vi "COM.vi"() -> ()   [LabVIEW 2013]
uses:
  <vilib>/Utility/file.llb/Write To Spreadsheet File (DBL).vi
panel:
  in  "Відстань \nреагування":dbl=30.0
  out "OloLo":bool
  out "Відстань в см.":dbl
  in  "Шлях для збереження даних в файл":path=path "C:/ULTRA/COM/first.csv"
  out "Посилка":i32
  in  "stop":bool
  out "Отриманий текст":string
  in  "Вибір порта для\n отримання даних":refnum<visa-resource-name>
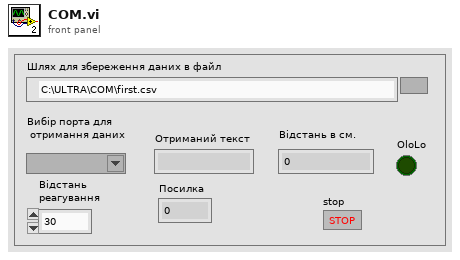
[diagram p1: front panel]
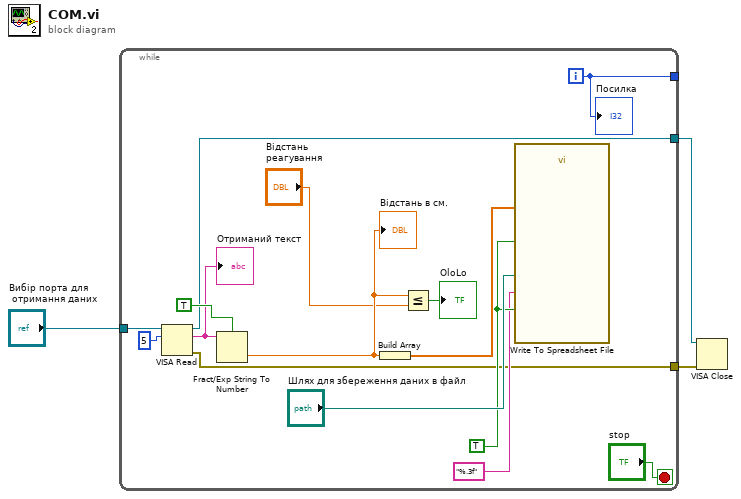
[diagram p0: block diagram]
diagram:
  n1 = while {
    tunnel: "Вибір порта для\n отримання даних" -> [w18]
    tunnel: [w9] -> _
    tunnel: [w13] -> w2
    tunnel: [w7] -> w1
    i -> [w9]
    stop <- "stop" stop-if-true
    w11 = TRUE
    n2 = VISA Read(VISA resource name=w18, byte count=u32 5) -> (VISA resource name out=w13:refnum<visa-resource-name>, read buffer=w14:string, error out=w7:errorcluster)  [unwired: 1 in, 1 out]
    "Отриманий текст" <- w14
    n3 = Fract/Exp String To Number(use system decimal point (T)=TRUE, string=w14) -> (number=w5:dbl)  [unwired: 2 in, 1 out]
    "Відстань в см." <- w5
    n4 = Build Array "Build Array"(w5) -> (w8:dbl[])
    n5 = Less Or Equal?(x=w5, y="Відстань \nреагування") -> (x <= y?=→"OloLo":bool)
    n6 = call-poly <vilib>:"Write To Spreadsheet File.vi"("transpose? (no:F)"=w11, "format (%.3f)"="%.3f", "append to file? (new file:F)"=w11, "1D data"=w8, "file path (dialog if empty)"="Шлях для збереження даних в файл") -> ()  [unwired: 3 in, 1 out]
    "Посилка" <- w9
  }
  n7 = VISA Close(VISA resource name=w2, error in (no error)=w1) -> ()  [unwired: 1 out]
